vi "Create Random Trial Array.vi"(10 "Trials":i32, 11 "Random Trials":bool) -> (3 "Trials Array":i32[](array[numeric]))   [LabVIEW 2013]
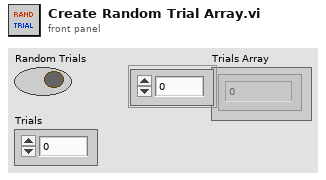
[diagram p1: front panel]
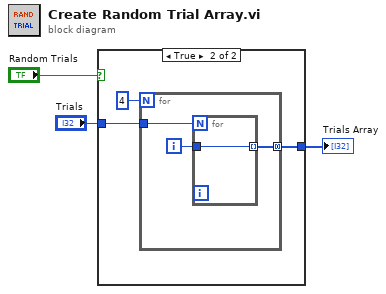
[diagram p0: block diagram]
diagram:
  n1 = case shown="True" "Random Trials" {
    tunnel: "Trials" -> [_ w5]
    tunnel: [_ w4] -> w2
    frame False {
    }
    frame True {
      n2 = for {
        N: 4 ("Conditions") -> [_]
        tunnel: [w8] -> w4 mode=concatenating
        tunnel: w5 -> [w7]
        i -> [w9]
        n3 = for {
          N: w7 -> [_]
          tunnel: w9 -> [w10]
          tunnel: [w10] -> w8 mode=indexing
        }
      }
    }
  }
  "Trials Array" <- w2
